vi "Write 3458_Config.vi"(8 "error in (no error)":errorcluster, 10 "clAnalysisConfig":T1={"HP 3458 address"="", "Amplitude"=0.0, "3458  Params:"={"Record Size"=4096, "Input Freq (Hz)"=50.0, "# Cycles (Desired)"=501.0, "Sampling Mode:"=1, "# of Record Avgs./Meas."=1, "Trigger Mode"=0, "Trig. Level (%)"=0.0, "# of Meas. Runs"=5, "Trigger Slope"=0}} {"3458  Params:"."Sampling Mode:" items=["DCV", "DCV (Corrected)", "DSDC", "SSDC"]; "3458  Params:"."Trigger Mode" items=["LEVEL", "EXTERNAL"]; "3458  Params:"."Trigger Slope" items=["POSITIVE", "NEGATIVE"]}, 11 "CorrFactor in":refnum<class "CorrFactor.lvclass">) -> (0 "error out":errorcluster, 3 "CorrFactor out":refnum<class "CorrFactor.lvclass">)   [LabVIEW 2018, in "AnalysisPlugins.lvlib" / "CorrFactor.lvclass"]
uses:
  CorrFactor.lvclass
  Typedefs/clAnalysisConfig.ctl
  Typedefs/3458 Params.ctl
  CorrFactor.lvclass/CorrFactor.ctl
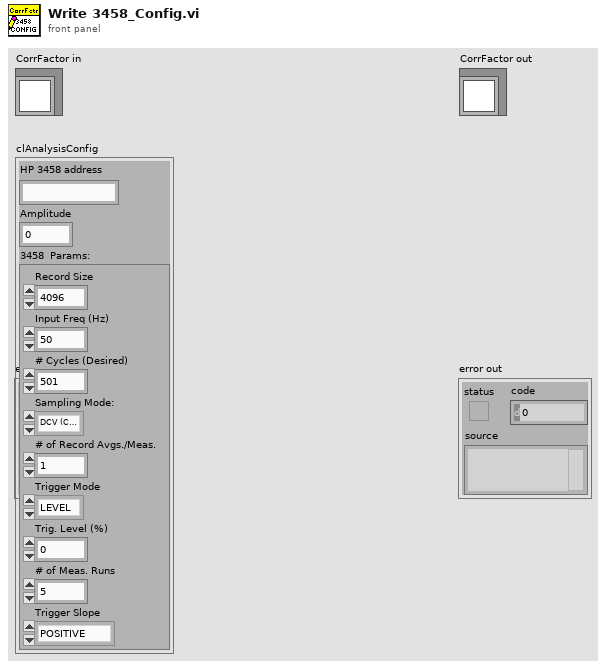
[diagram p1: front panel]
types:
  T1 = typedef "AnalysisPlugins.lvlib/CorrFactor.lvclass/clAnalysisConfig.ctl" = cluster{"HP 3458 address":string, "Amplitude":dbl, "3458  Params:":T2}
  T2 = typedef "AnalysisPlugins.lvlib/CorrFactor.lvclass/3458 Params.ctl" = cluster{"Record Size":i32, "Input Freq (Hz)":dbl, "# Cycles (Desired)":dbl, "Sampling Mode:":u16, "# of Record Avgs./Meas.":i32, "Trigger Mode":u16, "Trig. Level (%)":dbl, "# of Meas. Runs":i32, "Trigger Slope":u16}
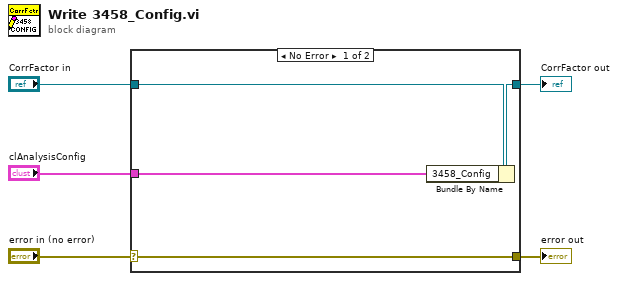
[diagram p0: block diagram]
diagram:
  n1 = case shown="No Error" "error in (no error)" {
    selector: "error in (no error)" -> [w9 w10]
    tunnel: [w9 w10] -> w4
    tunnel: [w7 w11] -> w2
    tunnel: "CorrFactor in" -> [w8 w11]
    tunnel: "clAnalysisConfig" -> [w6 _]
    frame No Error {
      n2 = Bundle By Name(cluster=w8, "3458_Config"=w6) -> (w7:refnum<class "CorrFactor.lvclass">)
    }
    frame Error {
    }
  }
  "error out" <- w4
  "CorrFactor out" <- w2
